vi "Get Data from RAM.vi"(8 "error in (no error)":errorcluster, 9 "End offset":u64, 10 "Start offset":u64, 11 "RP Communicator in":refnum<class "RP Communicator.lvclass">) -> (0 "error out":errorcluster, 2 "data out":string, 3 "RP Communicator out":refnum<class "RP Communicator.lvclass">)   [LabVIEW 2021, in "RP Communicator.lvclass"]
uses:
  RP Communicator.lvclass
  RP Command.ctl
  RP Communicator.lvclass/RP Communicator.ctl
  RP Write Command TCP.vi
panel:
  out "attempts":i32
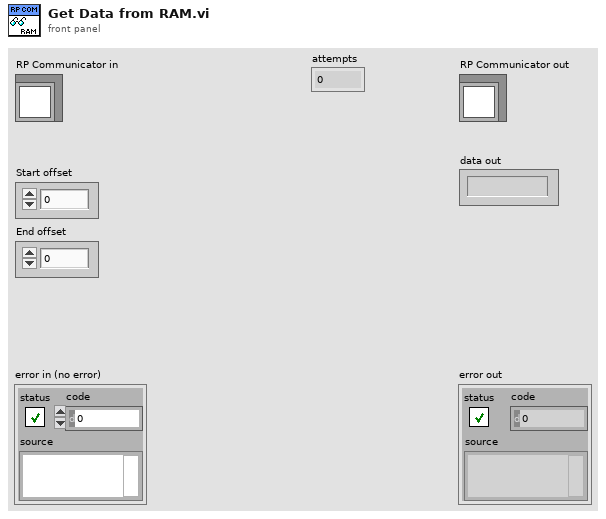
[diagram p1: front panel]
types:
  T1 = typedef "RP Command.ctl" = enum16{"Reset", "Read IDN", "Stop server", "Get status", "Get temperature", "Connect client", "Arm", "Software trigger", "Get whole buffer", "Get chunk", "System call", "Get config", "Set config", "Recieve data", "Recieve Calibartion", "Transmit data"}
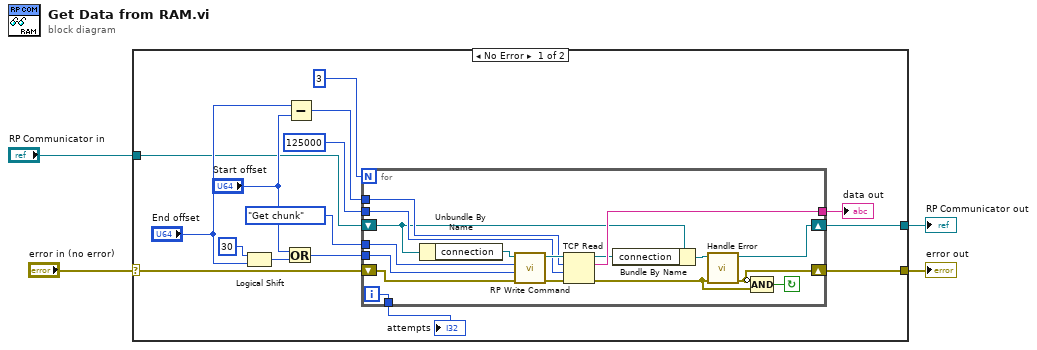
[diagram p0: block diagram]
diagram:
  n1 = case shown="No Error" "error in (no error)" {
    selector: "error in (no error)" -> [w11 w38]
    tunnel: [w10 w38] -> w3
    tunnel: [w6 w37] -> w1
    tunnel: "RP Communicator in" -> [w7 w37]
    frame No Error {
      n2 = Logical Shift(y=i16 30, x="End offset") -> (x << y=w17:u64)
      n3 = Or(x="Start offset", y=w17) -> (x .or. y?=w16:u64)
      n4 = Subtract(x="End offset", y="Start offset") -> (x-y=w13:u64)
      n5 = for {
        N: 3 -> [_]
        tunnel: RP_Command."Get chunk" ("Command number") -> [w34]
        tunnel: w16 -> [w33]
        tunnel: w13 -> [w32]
        tunnel: 125000 ("timeout ms (25000)") -> [w31]
        tunnel: [w29] -> w9
        shift-right: [w24] -> w6
        shift-left: w7 -> [w26]
        shift-right: [w22] -> w10
        shift-left: w11 -> [w30]
        tunnel: [w20] -> w5
        i -> [w20]
        stop <- w21 continue-if-true
        n6 = Unbundle By Name(w26) -> ("connection"=w28:refnum<k5>)
        n7 = call-poly "RP Write Command.vi"("Error In"=w30, "Command payload"=w33, "Command number"=w34, "connection ID"=w28) -> ("Error Out"=w36:errorcluster, "connection ID out"=w35:refnum<k5>)  [unwired: 5 in, 1 out]
        n8 = TCP Read(connection ID=w35, bytes to read=w32, error in (no error)=w36, 9:w31) -> (connection ID out=w27:refnum<k5>, data out=w29:string, error out=w23:errorcluster)  [unwired: 1 in]
        n9 = Bundle By Name(cluster=w26, "connection"=w27) -> (w25:refnum<class "RP Communicator.lvclass">)
        n10 = call-dynamic "Handle Error.vi"("error in (no error)"=w23, "RP Communicator in"=w25) -> ("error out"=w22:errorcluster, "RP Communicator out"=w24:refnum<class "RP Communicator.lvclass">)  [unwired: 8 in]
        n11 = Compound Arithmetic op=AND(invert w22, w23) -> (w21:bool)
      }
      "data out" <- w9
      "attempts" <- w5
    }
    frame Error {
    }
  }
  "error out" <- w3
  "RP Communicator out" <- w1
